vi "DL-Open Data Log.vi"(0 "Path":path) -> (4 "Header":T1, 15 "error out":errorcluster)   [LabVIEW 2015]
uses:
  Typedefs/DL-File Header.ctl
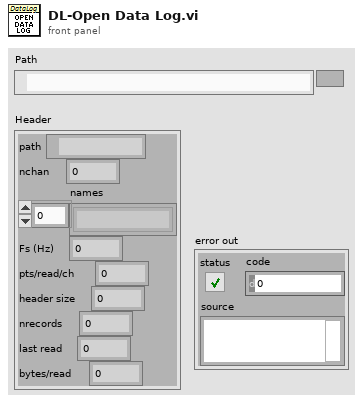
[diagram p1: front panel]
types:
  T1 = typedef "DL-File Header.ctl" = cluster{"path":path, "nchan":i32, "names":string[], "Fs (Hz)":dbl, "pts/read/ch":i32, "header size":i32, "nrecords":i32, "last read":i32, "bytes/read":i32}
  T2 = enum16{"open", "replace", "create", "open or create", "replace or create", "replace or create with confirmation"}
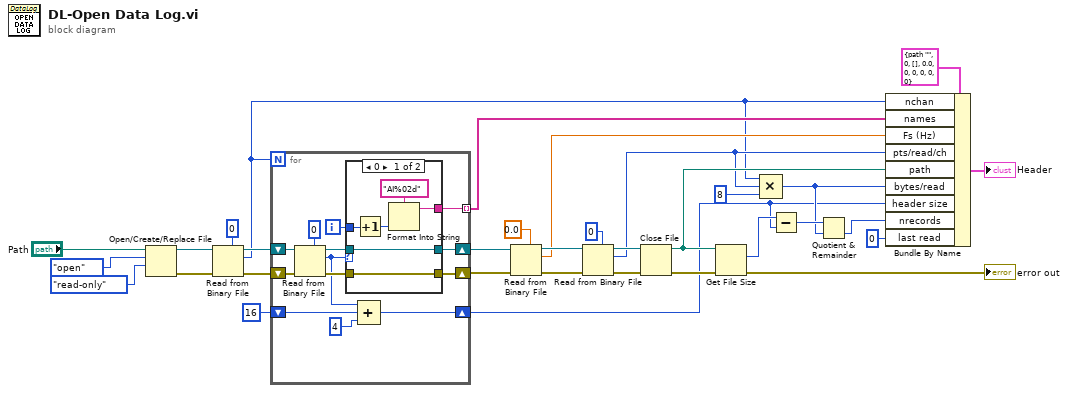
[diagram p0: block diagram]
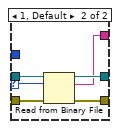
[diagram p2: hidden frame]
diagram:
  n1 = Open/Create/Replace File(file path (use dialog)="Path", operation (0:open)=T2."open", access (0:read/write)=enum16{"read/write", "read-only", "write-only"}."read-only") -> (refnum out=w29:refnum<file>, error out=w28:errorcluster)  [unwired: 3 in, 1 out]
  n2 = Read from Binary File(5:0, 8:w28, 11:w29) -> (0:w25:errorcluster, 2:w3:i32, 3:w24:refnum<file>)  [unwired: 3 in, 1 out]
  n3 = for {
    N: w3 -> [_]
    shift-right: [w42] -> w21
    shift-left: w24 -> [w46]
    shift-right: [w41] -> w20
    shift-left: w25 -> [w45]
    shift-right: [w36] -> w1
    shift-left: 16 -> [w39]
    tunnel: [w34] -> w22 mode=indexing
    i -> [w35]
    n4 = Read from Binary File(5:0, 8:w45, 11:w46) -> (0:w40:errorcluster, 2:w37:i32, 3:w43:refnum<file>)  [unwired: 3 in, 1 out]
    n5 = case shown="0" w37 {
      selector: w37 -> [_ w56]
      tunnel: w43 -> [w52 w58]
      tunnel: [w52 w55] -> w42
      tunnel: [w51 w54] -> w41
      tunnel: w40 -> [w51 w57]
      tunnel: w35 -> [w49 _]
      tunnel: [w48 w53] -> w34
      frame 0 {
        n6 = Increment(x=w49) -> (x+1=w50:i32)
        n7 = Format Into String(format string="AI%02d", w50) -> (resulting string=w48:string)  [unwired: 2 in, 1 out]
      }
      frame 1, Default {
        n8 = Read from Binary File(8:w57, 10:w56, 11:w58) -> (0:w54:errorcluster, 2:w53:string, 3:w55:refnum<file>)  [unwired: 3 in, 1 out]
      }
    }
    n9 = Compound Arithmetic op=ADD(w37, w39, 4 ("y")) -> (w36:i32)
  }
  n10 = Read from Binary File(5:0.0, 8:w20, 11:w21) -> (0:w18:errorcluster, 2:w16:dbl, 3:w19:refnum<file>)  [unwired: 3 in, 1 out]
  n11 = Read from Binary File(5:0, 8:w18, 11:w19) -> (0:w13:errorcluster, 2:w5:i32, 3:w14:refnum<file>)  [unwired: 3 in, 1 out]
  n12 = Close File(refnum=w14, error in=w13) -> (path=w11:path, error out=w10:errorcluster)
  n13 = Get File Size(file=w11, error in=w10) -> (size (in bytes)=w8:i64, 0:→"error out":errorcluster)  [unwired: 1 out]
  n14 = Compound Arithmetic op=MULTIPLY(w3, w5, 8 ("value")) -> (w2:i32)
  n15 = Subtract(x=w8, y=w1) -> (x-y=w6:i64)
  n16 = Quotient & Remainder(x=w6, y=w2) -> (floor(x/y)=w7:i64)  [unwired: 1 out]
  n17 = Bundle By Name(cluster=T1 {"path"=path "", "nchan"=0, "names"=[], "Fs (Hz)"=0.0, "pts/read/ch"=0, "header size"=0, "nrecords"=0, "last read"=0, "bytes/read"=0} ("Header"), "nchan"=w3, "names"=w22, "Fs (Hz)"=w16, "pts/read/ch"=w5, "path"=w11, "bytes/read"=w2, "header size"=w1, "nrecords"=w7, "last read"=0) -> (→"Header":T1)
